vi "loseq.vi"() -> ()   [LabVIEW 2013]
uses:
  <vilib>/NI/Tag Bus/table/data table.ctl
  <vilib>/NI/Tag Bus/table/transfer specification.ctl
  <vilib>/NI/Tag Bus/tag/Data Type.ctl
  <vilib>/Platform/TimedLoop/XDataNode/timing_clust.ctl
  <vilib>/Platform/TimedLoop/XDataNode/nitl_modes.ctl
  <vilib>/Platform/TimedLoop/XDataNode/wakeup.ctl
  <vilib>/platform/TimedLoop/XDataNode/XDataNode.xnode
  <vilib>/NI/Tag Bus/table/data table.lvlib
  <vilib>/Platform/TimedLoop/XDataNode/XDNodeRunTimeDep.lvlib
  <vilib>/NI/Tag Bus/tag/tag descriptor.lvclass
panel:
  out "dt":dbl
  in  "bad?":bool
  out "input data":T1
  out "data table sink out":T1
  out "error out":errorcluster
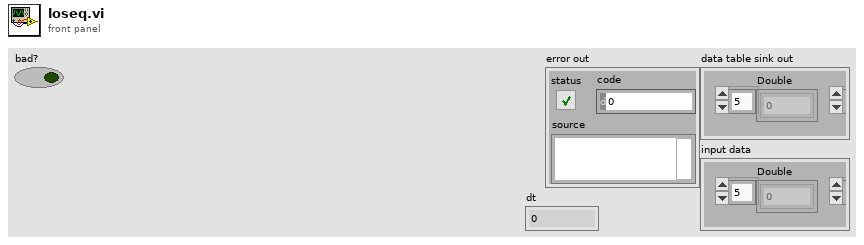
[diagram p1: front panel]
types:
  T1 = typedef "tag bus.lvlib/data table.lvlib/data table.ctl" = cluster{"Double":dbl[], "Single":sgl[], "I64":i64[], "I32":i32[], "I16":i16[], "I8":i8[], "U64":u64[], "U32":u32[], "U16":u16[], "U8":u8[], "Boolean":bool[], "String":string[], "Array of Double":cluster{"DBL Array":dbl[]}[], "Array of Single":cluster{"SGL Array":sgl[]}[], "Array of I64":cluster{"I64 Array":i64[]}[], "Array of I32":cluster{"I32 Array":i32[]}[], "Array of I16":cluster{"I16 Array":i16[]}[], "Array of I8":cluster{"I8 Array":i8[]}[], "Array of U64":cluster{"U64 Array":u64[]}[], "Array of U32":cluster{"U32 Array":u32[]}[], "Array of U16":cluster{"U16 Array":u16[]}[], "Array of U8":cluster{"U8 Array":u8[]}[], "Array of Boolean":cluster{"Boolean Array":bool[]}[], "Array of String":cluster{"String Array":string[]}[]}
  T2 = typedef "tag bus.lvlib/data table.lvlib/transfer specification.ctl" = cluster{"data type":T3, "sink indices":i32[], "source indices":i32[]}
  T3 = typedef "tag bus.lvlib/tag descriptor.lvclass/Data Type.ctl" = enum16{"Double", "Single", "I64", "I32", "I16", "I8", "U64", "U32", "U16", "U8", "Boolean", "String", "Array of Double", "Array of Single", "Array of I64", "Array of I32", "Array of I16", "Array of I8", "Array of U64", "Array of U32", "Array of U16", "Array of U8", "Array of Boolean", "Array of String"}
  T4 = typedef "XDNodeRunTimeDep.lvlib/timing_clust.ctl" = cluster{"Expected End [f-1]":u64, "Actual End [f-1]":u64, "Finished Late? [f-1]":bool, "Expected End [i-1]":u64, "Actual End [i-1]":u64, "Finished Late? [i-1]":bool, "Expected Start [i]":u64, "Actual Start [i]":u64, "Expected Start [f]":u64, "Actual Start [f]":u64, "Source Name":string, "Structure Name":string, "Period":i64, "Deadline":i64, "Offset":i64, "Start":i64, "Priority":i32, "Timeout":i32, "Mode":T5, "Wakeup Reason":T6, "Error":errorcluster, "Source Type":string, "Secondary Source Type":string, "Global End Time":u64, "Global Start Time":u64, "Frame Duration":u64, "Iteration Duration":u64, "Assigned CPU":i32, "I/O Scan Engine Mode":u32}
  T5 = typedef "XDNodeRunTimeDep.lvlib/nitl_modes.ctl" = enum32{"No Change", "Process missed periods, maintain original phase", "Discard missed periods, maintain original phase", "Process missed periods, ignore original phase", "Discard missed periods, ignore original phase"}
  T6 = typedef "XDNodeRunTimeDep.lvlib/wakeup.ctl" = enum32{"Normal", "Aborted", "Asynchronous wakeup", "Timing source error", "Timed loop error", "Timeout"}
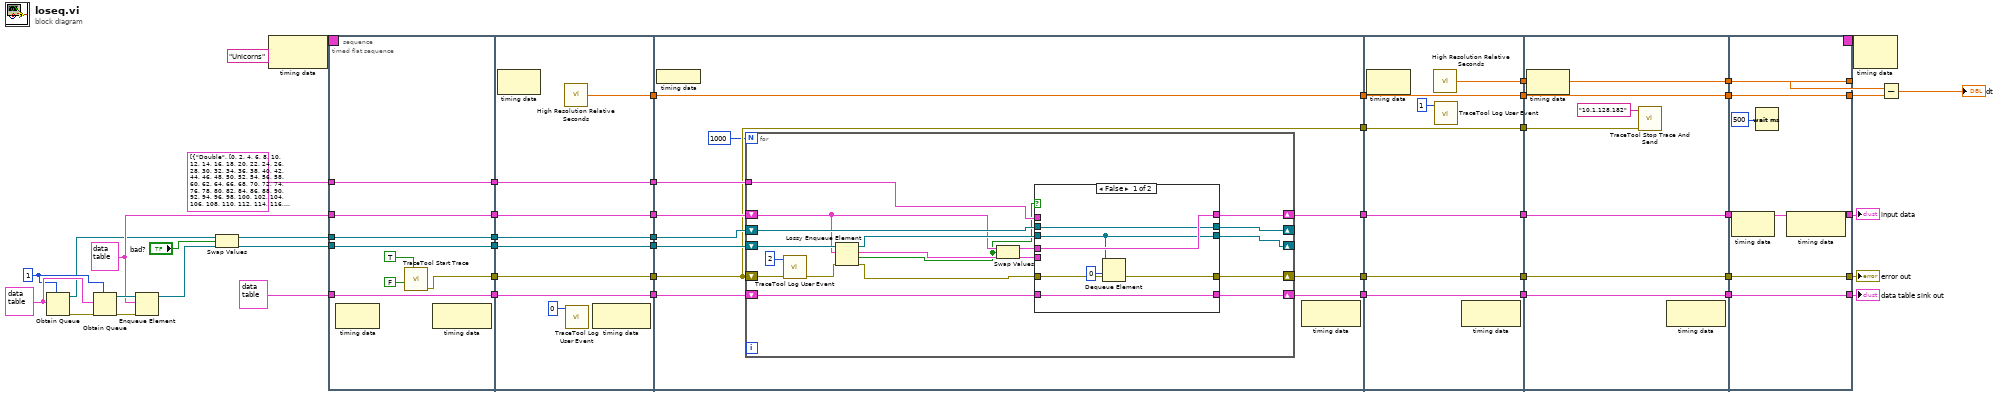
[diagram p0: block diagram]
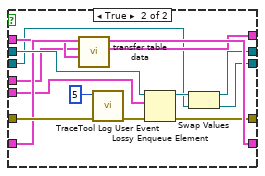
[diagram p2: hidden frame]
diagram:
  w12 = T1 {"Double"=[22.0, 22.0, 22.0, 22.0, 22.0, 22.0, 22.0, 22.0, 22.0, 22.0, 22.0, 22.0, 22.0, 22.0, 22.0, 22.0, 22.0, 22.0, 22.0, 22.0, 22.0, 22.0, 22.0, 22.0, 22.0, 22.0, 22.0, 22.0, 22.0, 22.0, 22.0, 22.0, 22.0, 22.0, 22.0, 22.0, 22.0, 22.0, 22.0, 22.0, 22.0, 22.0, 22.0, 22.0, 22.0, 22.0, 22.0, 22.0, 22.0, 22.0, 22.0, 22.0, 22.0, 22.0, 22.0, 22.0, 22.0, 22.0, 22.0, 22.0, 22.0, 22.0, 22.0, 22.0, 22.0, 22.0, 22.0, 22.0, 22.0, 22.0, 22.0, 22.0, 22.0, 22.0, 22.0, 22.0, 22.0, 22.0, 22.0, 22.0, 22.0, 22.0, 22.0, 22.0, 22.0, 22.0, 22.0, 22.0, 22.0, 22.0, 22.0, 22.0, 22.0, 22.0, 22.0, 22.0, 22.0, 22.0, 22.0, 22.0, 22.0, 22.0, 22.0, 22.0, 22.0, 22.0, 22.0, 22.0, 22.0, 22.0, 22.0, 22.0, 22.0, 22.0, 22.0, 22.0, 22.0, 22.0, 22.0, 22.0, 22.0, 22.0, 22.0, 22.0, 22.0, 22.0, 22.0, 22.0, 22.0, 22.0, 22.0, 22.0, 22.0, 22.0, 22.0, 22.0, 22.0, 22.0, 22.0, 22.0, 22.0, 22.0, 22.0, 22.0, 22.0, 22.0, 22.0, 22.0, 22.0, 22.0, 22.0, 22.0, 22.0, 22.0, 22.0, 22.0, 22.0, 22.0, 22.0, 22.0, 22.0, 22.0, 22.0, 22.0, 22.0, 22.0, 22.0, 22.0, 22.0, 22.0, 22.0, 22.0, 22.0, 22.0, 22.0, 22.0, 22.0, 22.0, 22.0, 22.0, 22.0, 22.0, 22.0, 22.0, 22.0, 22.0, 22.0, 22.0, 22.0, 22.0, 22.0, 22.0, 22.0, 22.0, 22.0, 22.0, 22.0, 22.0, 22.0, 22.0, 22.0, 22.0, 22.0, 22.0, 22.0, 22.0, 22.0, 22.0, 22.0, 22.0, 22.0, 22.0, 22.0, 22.0, 22.0, 22.0, 22.0, 22.0, 22.0, 22.0, 22.0, 22.0, 22.0, 22.0, 22.0, 22.0, 22.0, 22.0, 22.0, 22.0, 22.0, 22.0, 22.0, 22.0, 22.0, 22.0, 22.0, 22.0, 22.0, 22.0, 22.0, 22.0, 22.0, 22.0, 22.0, 22.0, 22.0, 22.0, 22.0, 22.0, 22.0, 22.0, 22.0, 22.0, 22.0, 22.0, 22.0, 22.0, 22.0, 22.0, 22.0, 22.0, 22.0, 22.0, 22.0, 22.0, 22.0, 22.0, 22.0, 22.0, 22.0, 22.0, 22.0, 22.0, 22.0, 22.0, 22.0, 22.0, 22.0, 22.0, 22.0, 22.0, 22.0, 22.0, 22.0, 22.0, 22.0, 22.0, 22.0, 22.0, 22.0, 22.0, 22.0, 22.0, 22.0, 22.0, 22.0, 22.0, 22.0, 22.0, 22.0, 22.0, 22.0, 22.0, 22.0, 22.0, 22.0, 22.0, 22.0, 22.0, 22.0, 22.0, 22.0, 22.0, 22.0, 22.0, 22.0, 22.0, 22.0, 22.0, 22.0, 22.0, 22.0, 22.0, 22.0, 22.0, 22.0, 22.0, 22.0, 22.0, 22.0, 22.0, 22.0, 22.0, 22.0, 22.0, 22.0, 22.0, 22.0, 22.0, 22.0, 22.0, 22.0, 22.0, 22.0, 22.0, 22.0, 22.0, 22.0, 22.0, 22.0, 22.0, 22.0, 22.0, 22.0, 22.0, 22.0, 22.0, 22.0, 22.0, 22.0, 22.0, 22.0, 22.0, 22.0, 22.0, 22.0, 22.0, 22.0, 22.0, 22.0, 22.0, 22.0, 22.0, 22.0, 22.0, 22.0, 22.0, 22.0, 22.0, 22.0, 22.0, 22.0, 22.0, 22.0, 22.0, 22.0, 22.0, 22.0, 22.0, 22.0, 22.0, 22.0, 22.0, 22.0, 22.0, 22.0, 22.0, 22.0, 22.0, 22.0, 22.0, 22.0, 22.0, 22.0, 22.0, 22.0, 22.0, 22.0, 22.0, 22.0, 22.0, 22.0, 22.0, 22.0, 22.0, 22.0, 22.0, 22.0, 22.0, 22.0, 22.0, 22.0, 22.0, 22.0, 22.0, 22.0, 22.0, 22.0, 22.0, 22.0, 22.0, 22.0, 22.0, 22.0, 22.0, 22.0, 22.0, 22.0, 22.0, 22.0, 22.0, 22.0, 22.0, 22.0, 22.0, 22.0, 22.0, 22.0, 22.0, 22.0, 22.0, 22.0, 22.0, 22.0, 22.0, 22.0, 22.0, 22.0, 22.0, 22.0, 22.0, 22.0, 22.0, 22.0, 22.0, 22.0, 22.0, 22.0, 22.0, 22.0, 22.0, 22.0, 22.0, 22.0, 22.0, 22.0, 22.0, 22.0, 22.0, 22.0, 22.0, 22.0, 22.0, 22.0, 22.0, 22.0, 22.0, 22.0, 22.0, 22.0, 22.0, 22.0, 22.0, 22.0, 22.0, 22.0, 22.0, 22.0, 22.0], "Single"=[], "I64"=[], "I32"=[], "I16"=[], "I8"=[], "U64"=[], "U32"=[], "U16"=[], "U8"=[], "Boolean"=[], "String"=[], "Array of Double"=[], "Array of Single"=[], "Array of I64"=[], "Array of I32"=[], "Array of I16"=[], "Array of I8"=[], "Array of U64"=[], "Array of U32"=[], "Array of U16"=[], "Array of U8"=[], "Array of Boolean"=[], "Array of String"=[]} ("output cluster 2")
  w21 = 1 ("max queue size (-1, unlimited)")
  w22 = T1 {"Double"=[], "Single"=[], "I64"=[], "I32"=[], "I16"=[], "I8"=[], "U64"=[], "U32"=[], "U16"=[], "U8"=[], "Boolean"=[], "String"=[], "Array of Double"=[], "Array of Single"=[], "Array of I64"=[], "Array of I32"=[], "Array of I16"=[], "Array of I8"=[], "Array of U64"=[], "Array of U32"=[], "Array of U16"=[], "Array of U8"=[], "Array of Boolean"=[], "Array of String"=[]} ("input data")
  n1 = Obtain Queue(max queue size (-1, unlimited)=w21, element data type=w22) -> (queue out=w9:refnum<queue>, error out=w18:errorcluster)  [unwired: 3 in, 1 out]
  n2 = Obtain Queue(max queue size (-1, unlimited)=w21, element data type=w22, error in (no error)=w18) -> (queue out=w16:refnum<queue>, error out=w17:errorcluster)  [unwired: 2 in, 1 out]
  n3 = Enqueue Element(queue=w16, element=w12, error in (no error)=w17) -> (queue out=w7:refnum<queue>)  [unwired: 1 in, 2 out]
  n4 = Swap Values(12:w9, 13:"bad?", 14:w7) -> (1:w8:refnum<queue>, 3:w6:refnum<queue>)
  n5 = node-c288("Unicorns" ("Structure Name")) -> (w20:T4)
  n6 = timed-sequence {
    timing: w20 -> [_]
    timing-out: [_] -> w19
    tunnel: w6 -> [w61]
    tunnel: w8 -> [w60]
    tunnel: [w59] -> w15
    tunnel: T1 {"Double"=array[1000 elements], "Single"=[], "I64"=[], "I32"=[], "I16"=[], "I8"=[], "U64"=[], "U32"=[], "U16"=[], "U8"=[], "Boolean"=[], "String"=[], "Array of Double"=[], "Array of Single"=[], "Array of I64"=[], "Array of I32"=[], "Array of I16"=[], "Array of I8"=[], "Array of U64"=[], "Array of U32"=[], "Array of U16"=[], "Array of U8"=[], "Array of Boolean"=[], "Array of String"=[]} ("output cluster") -> [w58]
    tunnel: [w57] -> w13
    tunnel: w12 -> [w56]
    tunnel: [w55] -> w11
    tunnel: T2[] [{"data type"=enum."Double", "sink indices"=[0, 2, 4, 6, 8, 10, 12, 14, 16, 18, 20, 22, 24, 26, 28, 30, 32, 34, 36, 38, 40, 42, 44, 46, 48, 50, 52, 54, 56, 58, 60, 62, 64, 66, 68, 70, 72, 74, 76, 78, 80, 82, 84, 86, 88, 90, 92, 94, 96, 98, 100, 102, 104, 106, 108, 110, 112, 114, 116, 118, 120, 122, 124, 126, 128, 130, 132, 134, 136, 138, 140, 142, 144, 146, 148, 150, 152, 154, 156, 158, 160, 162, 164, 166, 168, 170, 172, 174, 176, 178, 180, 182, 184, 186, 188, 190, 192, 194, 196, 198, 200, 202, 204, 206, 208, 210, 212, 214, 216, 218, 220, 222, 224, 226, 228, 230, 232, 234, 236, 238, 240, 242, 244, 246, 248, 250, 252, 254, 256, 258, 260, 262, 264, 266, 268, 270, 272, 274, 276, 278, 280, 282, 284, 286, 288, 290, 292, 294, 296, 298, 300, 302, 304, 306, 308, 310, 312, 314, 316, 318, 320, 322, 324, 326, 328, 330, 332, 334, 336, 338, 340, 342, 344, 346, 348, 350, 352, 354, 356, 358, 360, 362, 364, 366, 368, 370, 372, 374, 376, 378, 380, 382, 384, 386, 388, 390, 392, 394, 396, 398, 400, 402, 404, 406, 408, 410, 412, 414, 416, 418, 420, 422, 424, 426, 428, 430, 432, 434, 436, 438, 440, 442, 444, 446, 448, 450, 452, 454, 456, 458, 460, 462, 464, 466, 468, 470, 472, 474, 476, 478, 480, 482, 484, 486, 488, 490, 492, 494, 496, 498, 500, 502, 504, 506, 508, 510, 512, 514, 516, 518, 520, 522, 524, 526, 528, 530, 532, 534, 536, 538, 540, 542, 544, 546, 548, 550, 552, 554, 556, 558, 560, 562, 564, 566, 568, 570, 572, 574, 576, 578, 580, 582, 584, 586, 588, 590, 592, 594, 596, 598, 600, 602, 604, 606, 608, 610, 612, 614, 616, 618, 620, 622, 624, 626, 628, 630, 632, 634, 636, 638, 640, 642, 644, 646, 648, 650, 652, 654, 656, 658, 660, 662, 664, 666, 668, 670, 672, 674, 676, 678, 680, 682, 684, 686, 688, 690, 692, 694, 696, 698, 700, 702, 704, 706, 708, 710, 712, 714, 716, 718, 720, 722, 724, 726, 728, 730, 732, 734, 736, 738, 740, 742, 744, 746, 748, 750, 752, 754, 756, 758, 760, 762, 764, 766, 768, 770, 772, 774, 776, 778, 780, 782, 784, 786, 788, 790, 792, 794, 796, 798, 800, 802, 804, 806, 808, 810, 812, 814, 816, 818, 820, 822, 824, 826, 828, 830, 832, 834, 836, 838, 840, 842, 844, 846, 848, 850, 852, 854, 856, 858, 860, 862, 864, 866, 868, 870, 872, 874, 876, 878, 880, 882, 884, 886, 888, 890, 892, 894, 896, 898, 900, 902, 904, 906, 908, 910, 912, 914, 916, 918, 920, 922, 924, 926, 928, 930, 932, 934, 936, 938, 940, 942, 944, 946, 948, 950, 952, 954, 956, 958, 960, 962, 964, 966, 968, 970, 972, 974, 976, 978, 980, 982, 984, 986, 988, 990, 992, 994, 996, 998], "source indices"=[0, 1, 2, 3, 4, 5, 6, 7, 8, 9, 10, 11, 12, 13, 14, 15, 16, 17, 18, 19, 20, 21, 22, 23, 24, 25, 26, 27, 28, 29, 30, 31, 32, 33, 34, 35, 36, 37, 38, 39, 40, 41, 42, 43, 44, 45, 46, 47, 48, 49, 50, 51, 52, 53, 54, 55, 56, 57, 58, 59, 60, 61, 62, 63, 64, 65, 66, 67, 68, 69, 70, 71, 72, 73, 74, 75, 76, 77, 78, 79, 80, 81, 82, 83, 84, 85, 86, 87, 88, 89, 90, 91, 92, 93, 94, 95, 96, 97, 98, 99, 100, 101, 102, 103, 104, 105, 106, 107, 108, 109, 110, 111, 112, 113, 114, 115, 116, 117, 118, 119, 120, 121, 122, 123, 124, 125, 126, 127, 128, 129, 130, 131, 132, 133, 134, 135, 136, 137, 138, 139, 140, 141, 142, 143, 144, 145, 146, 147, 148, 149, 150, 151, 152, 153, 154, 155, 156, 157, 158, 159, 160, 161, 162, 163, 164, 165, 166, 167, 168, 169, 170, 171, 172, 173, 174, 175, 176, 177, 178, 179, 180, 181, 182, 183, 184, 185, 186, 187, 188, 189, 190, 191, 192, 193, 194, 195, 196, 197, 198, 199, 200, 201, 202, 203, 204, 205, 206, 207, 208, 209, 210, 211, 212, 213, 214, 215, 216, 217, 218, 219, 220, 221, 222, 223, 224, 225, 226, 227, 228, 229, 230, 231, 232, 233, 234, 235, 236, 237, 238, 239, 240, 241, 242, 243, 244, 245, 246, 247, 248, 249, 250, 251, 252, 253, 254, 255, 256, 257, 258, 259, 260, 261, 262, 263, 264, 265, 266, 267, 268, 269, 270, 271, 272, 273, 274, 275, 276, 277, 278, 279, 280, 281, 282, 283, 284, 285, 286, 287, 288, 289, 290, 291, 292, 293, 294, 295, 296, 297, 298, 299, 300, 301, 302, 303, 304, 305, 306, 307, 308, 309, 310, 311, 312, 313, 314, 315, 316, 317, 318, 319, 320, 321, 322, 323, 324, 325, 326, 327, 328, 329, 330, 331, 332, 333, 334, 335, 336, 337, 338, 339, 340, 341, 342, 343, 344, 345, 346, 347, 348, 349, 350, 351, 352, 353, 354, 355, 356, 357, 358, 359, 360, 361, 362, 363, 364, 365, 366, 367, 368, 369, 370, 371, 372, 373, 374, 375, 376, 377, 378, 379, 380, 381, 382, 383, 384, 385, 386, 387, 388, 389, 390, 391, 392, 393, 394, 395, 396, 397, 398, 399, 400, 401, 402, 403, 404, 405, 406, 407, 408, 409, 410, 411, 412, 413, 414, 415, 416, 417, 418, 419, 420, 421, 422, 423, 424, 425, 426, 427, 428, 429, 430, 431, 432, 433, 434, 435, 436, 437, 438, 439, 440, 441, 442, 443, 444, 445, 446, 447, 448, 449, 450, 451, 452, 453, 454, 455, 456, 457, 458, 459, 460, 461, 462, 463, 464, 465, 466, 467, 468, 469, 470, 471, 472, 473, 474, 475, 476, 477, 478, 479, 480, 481, 482, 483, 484, 485, 486, 487, 488, 489, 490, 491, 492, 493, 494, 495, 496, 497, 498, 499]}] ("appended array") -> [w54]
    tunnel: [w30] -> w4
    tunnel: [w29] -> w3
    n7 = timed-flat-sequence {
      tunnel: w56 -> [w66]
      tunnel: w58 -> [w67]
      tunnel: w60 -> [w68]
      tunnel: w61 -> [w69]
      tunnel: [w69] -> w53
      tunnel: [w68] -> w51
      tunnel: [w67] -> w49
      tunnel: [w66] -> w47
      tunnel: [w64] -> w45
      tunnel: w54 -> [w63]
      tunnel: [w63] -> w43
      tunnel: w53 -> [w79]
      tunnel: [w79] -> w52
      tunnel: w51 -> [w78]
      tunnel: [w78] -> w50
      tunnel: w49 -> [w77]
      tunnel: [w77] -> w48
      tunnel: w47 -> [w76]
      tunnel: [w76] -> w46
      tunnel: w45 -> [w75]
      tunnel: [w75] -> w44
      tunnel: w43 -> [w74]
      tunnel: [w74] -> w42
      tunnel: [w73] -> w32
      tunnel: [w87] -> w41
      tunnel: [w90] -> w39
      tunnel: [w89] -> w37
      tunnel: w52 -> [w85]
      tunnel: w50 -> [w92]
      tunnel: w48 -> [w91]
      tunnel: w46 -> [w86]
      tunnel: w44 -> [w83]
      tunnel: [w83] -> w35
      tunnel: w42 -> [w88]
      tunnel: [w84] -> w33
      tunnel: w32 -> [w84]
      tunnel: w41 -> [w141]
      tunnel: [w141] -> w40
      tunnel: w39 -> [w140]
      tunnel: [w140] -> w38
      tunnel: w37 -> [w139]
      tunnel: [w139] -> w36
      tunnel: w35 -> [w138]
      tunnel: [w138] -> w34
      tunnel: w33 -> [w137]
      tunnel: [w137] -> w31
      tunnel: [w136] -> w28
      tunnel: w40 -> [w150]
      tunnel: w38 -> [w149]
      tunnel: w36 -> [w148]
      tunnel: w34 -> [w147]
      tunnel: w31 -> [w145]
      tunnel: w28 -> [w144]
      tunnel: [w150] -> w27
      tunnel: [w149] -> w26
      tunnel: [w148] -> w25
      tunnel: [w145] -> w24
      tunnel: [w144] -> w23
      tunnel: [w154] -> w29
      tunnel: [w155] -> w30
      tunnel: [w156] -> w55
      tunnel: [w157] -> w57
      tunnel: [w158] -> w59
      tunnel: w27 -> [w158]
      tunnel: w26 -> [w157]
      tunnel: w25 -> [w156]
      tunnel: w24 -> [w155]
      tunnel: w23 -> [w154]
      frame #0 {
        n8 = node-c288() -> ()  [unwired: 1 in, 1 out]
        n9 = call <vilib>:"TraceTool Start Trace.vi"("Detailed Tracing? (F)"=TRUE, "VI Tracing? (T)"=FALSE) -> ("error out"=w64:errorcluster)  [unwired: 8 in, 1 out]
        n10 = node-c288() -> ()  [unwired: 1 in, 1 out]
      }
      frame #1 {
        n11 = node-c288() -> ()  [unwired: 1 in, 1 out]
        n12 = call <vilib>:"High Resolution Relative Seconds.vi"() -> ("relative seconds"=w73:dbl)
        n13 = call <vilib>:"TraceTool Log User Event.vi"("Event ID (0-255)"=u32 0) -> ()  [unwired: 10 in, 1 out]
        n14 = node-c288() -> ()  [unwired: 1 in, 1 out]
      }
      frame #2 {
        n15 = node-c288() -> ()  [unwired: 1 in]
        n16 = for {
          N: 1000 -> [_]
          tunnel: w88 -> [w107]
          shift-right: [w109] -> w90
          shift-left: w91 -> [w110]
          shift-right: [w108] -> w89
          shift-left: w86 -> [w95]
          shift-right: [w106] -> w87
          shift-left: w83 -> [w102]
          shift-right: [w104] -> _
          shift-left: w85 -> [w105]
          shift-right: [w103] -> _
          shift-left: w92 -> [w111]
          n17 = call <vilib>:"TraceTool Log User Event.vi"("error in (no error)"=w102, "Event ID (0-255)"=u32 2) -> ("error out"=w97:errorcluster)  [unwired: 9 in]
          n18 = Lossy Enqueue Element(queue=w105, element=w95, error in (no error)=w97) -> (queue out=w98:refnum<queue>, overflow element=w94:T1, overflow?=w93:bool, error out=w96:errorcluster)
          n19 = Swap Values(12:w95, 13:w93, 14:w94) -> (1:w100:T1, 3:w99:T1)
          n20 = case shown="False" w93 {
            tunnel: [w117 w132] -> w109
            tunnel: [w115 w131] -> w108
            tunnel: w96 -> [w116 w130]
            tunnel: [w116 w129] -> w106
            tunnel: w111 -> [w114 w128]
            tunnel: w110 -> [w117 w127]
            tunnel: w107 -> [_ w126]
            tunnel: w100 -> [w115 w125]
            tunnel: w99 -> [_ w124]
            tunnel: [w114 w122] -> w103
            tunnel: w98 -> [w113 w121]
            tunnel: [w113 w120] -> w104
            frame False {
              n21 = Dequeue Element(queue=w113, timeout in ms (-1)=0) -> ()  [unwired: 1 in, 4 out]
            }
            frame True {
              n22 = call <vilib>:"transfer table data.vi"("transfer specification in"=w126, "data table source in"=w125, "data table sink in"=w127) -> ("data table source out"=w131:T1, "data table sink out"=w132:T1)  [unwired: 6 in, 1 out]
              n23 = call <vilib>:"TraceTool Log User Event.vi"("error in (no error)"=w130, "Event ID (0-255)"=u32 5) -> ("error out"=w119:errorcluster)  [unwired: 9 in]
              n24 = Lossy Enqueue Element(queue=w128, element=w124, error in (no error)=w119) -> (queue out=w123:refnum<queue>, error out=w129:errorcluster)  [unwired: 2 out]
              n25 = Swap Values(12:w123, 14:w121) -> (1:w122:refnum<queue>, 3:w120:refnum<queue>)  [unwired: 1 in]
            }
          }
        }
        n26 = node-c288() -> ()  [unwired: 1 in, 1 out]
      }
      frame #3 {
        n27 = node-c288() -> ()  [unwired: 1 in, 1 out]
        n28 = call <vilib>:"High Resolution Relative Seconds.vi"() -> ("relative seconds"=w136:dbl)
        n29 = call <vilib>:"TraceTool Log User Event.vi"("Event ID (0-255)"=u32 1) -> ()  [unwired: 10 in, 1 out]
        n30 = node-c288() -> ()  [unwired: 1 in, 1 out]
      }
      frame #4 {
        n31 = node-c288() -> ()  [unwired: 1 in, 1 out]
        n32 = call <vilib>:"TraceTool Stop Trace And Send.vi"("error in (no error)"=w147, "Trace Host Network Address"="10.1.128.182") -> ()  [unwired: 9 in, 1 out]
        n33 = node-c288() -> ()  [unwired: 1 in, 1 out]
      }
      frame #5 {
        n34 = node-c288() -> ()  [unwired: 1 in, 1 out]
        n35 = Wait (ms)(milliseconds to wait=u32 500) -> ()  [unwired: 1 out]
        n36 = node-c288() -> ()  [unwired: 1 in, 1 out]
      }
    }
  }
  "error out" <- w15
  "data table sink out" <- w13
  "input data" <- w11
  n37 = node-c288(w19) -> ()  [unwired: 1 out]
  n38 = Subtract(x=w3, y=w4) -> (x-y=→"dt":dbl)
